vi "Initialize.vi"(8 "error in (no error)":errorcluster, 11 "Acquisition in":refnum<class "Acquisition.lvclass">) -> (0 "error out":errorcluster, 3 "Acquisition out":refnum<class "Acquisition.lvclass">)   [LabVIEW 2018, in "Acquisition.lvclass"]
uses:
  Acquisition.lvclass
  C:/Users/devstaff/sparc4/s4gui/Versao ZeroMQ REQ-REP/SPARC4_GUI -20241016_20241016/Server/Server.lvclass
  Server/Server.lvclass/Server.ctl
  Acquisition.lvclass/Acquisition.ctl
  Channel/Channel.lvclass/Channel.ctl
  Server/Server.lvclass
  Comm/Stream/Stream.lvclass
  Log/Log.lvclass
  Channel/Channel.lvclass
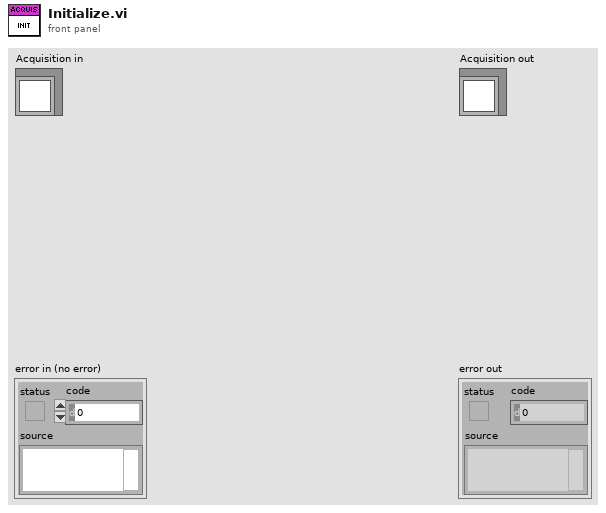
[diagram p1: front panel]
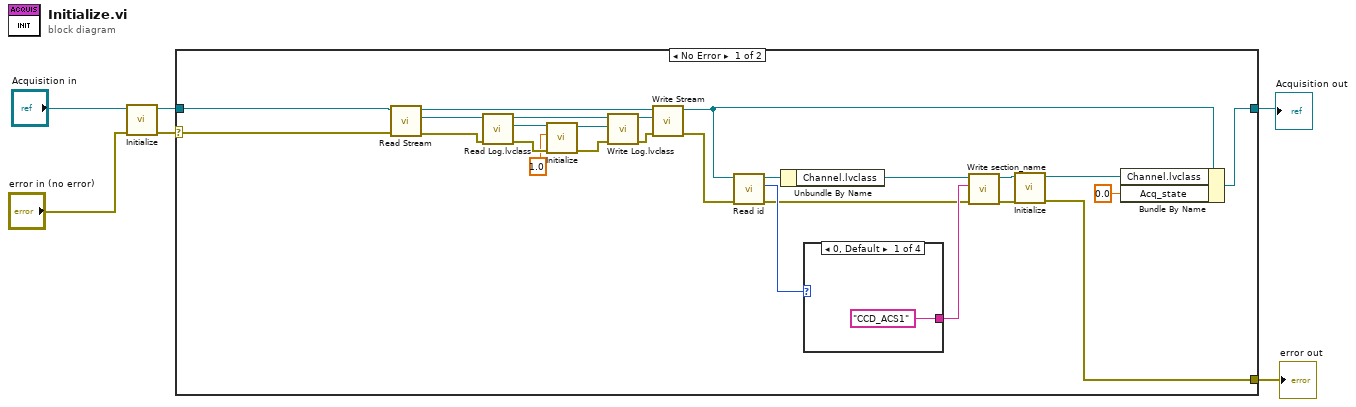
[diagram p0: block diagram]
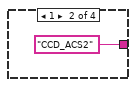
[diagram p2: hidden frame]
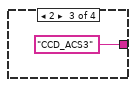
[diagram p3: hidden frame]
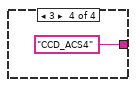
[diagram p4: hidden frame]
diagram:
  n1 = call-parent "Initialize.vi"("error in (no error)"="error in (no error)", "Server in"="Acquisition in") -> ("error out"=w1:errorcluster, "Server out"=w4:refnum<class "Acquisition.lvclass">)  [unwired: 8 in]
  n2 = case shown="No Error" w1 {
    selector: w1 -> [w11 w38]
    tunnel: [w31 w38] -> w3
    tunnel: [w8 w37] -> w2
    tunnel: w4 -> [w12 w37]
    frame No Error {
      n3 = call-dynamic "Read Stream.vi"("error in (no error)"=w11, "Server in"=w12) -> ("error out"=w9:errorcluster, "Stream.lvclass"=w10:refnum<class "Stream.lvclass">, "Server out"=w30:refnum<class "Acquisition.lvclass">)  [unwired: 7 in]
      n4 = call-dynamic "Read Log.lvclass.vi"("error in (no error)"=w9, "Comm in"=w10) -> ("error out"=w17:errorcluster, "Log.lvclass"=w19:refnum<class "Log.lvclass">, "Comm out"=w20:refnum<class "Stream.lvclass">)  [unwired: 7 in]
      n5 = call-dynamic "Initialize.vi"("error in (no error)"=w17, "Level"=1.0, "Log in"=w19) -> ("error out"=w16:errorcluster, "Log out"=w18:refnum<class "Log.lvclass">)  [unwired: 7 in]
      n6 = call-dynamic "Write Log.lvclass.vi"("error in (no error)"=w16, "Log.lvclass"=w18, "Comm in"=w20) -> ("error out"=w15:errorcluster, "Comm out"=w14:refnum<class "Stream.lvclass">)  [unwired: 7 in]
      n7 = call-dynamic "Write Stream.vi"("error in (no error)"=w15, "Stream.lvclass"=w14, "Server in"=w30) -> ("error out"=w22:errorcluster, "Server out"=w7:refnum<class "Acquisition.lvclass">)  [unwired: 7 in]
      n8 = call "Read id.vi"("error in (no error)"=w22, "Server in"=w7) -> ("error out"=w21:errorcluster, "id"=w27:u32, "Server out"=w28:refnum<class "Acquisition.lvclass">)  [unwired: 7 in]
      n9 = Unbundle By Name(w28) -> ("Channel.lvclass"=w26:refnum<class "Channel.lvclass">)
      n10 = case shown="0, Default" w27 {
        tunnel: ["CCD_ACS1" "CCD_ACS2" "CCD_ACS3" "CCD_ACS4"] -> w24
        frame 0, Default {
        }
        frame 1 {
        }
        frame 2 {
        }
        frame 3 {
        }
      }
      n11 = call "Write section_name.vi"("error in (no error)"=w21, "section_name"=w24, "Channel in"=w26) -> ("error out"=w23:errorcluster, "Channel out"=w25:refnum<class "Channel.lvclass">)  [unwired: 7 in]
      n12 = call-dynamic "Initialize.vi"("error in (no error)"=w23, "Channel in"=w25) -> ("error out"=w31:errorcluster, "Channel out"=w32:refnum<class "Channel.lvclass">)  [unwired: 8 in]
      n13 = Bundle By Name(cluster=w7, "Channel.lvclass"=w32, "Acq_state"=0.0) -> (w8:refnum<class "Acquisition.lvclass">)
    }
    frame Error {
    }
  }
  "Acquisition out" <- w2
  "error out" <- w3
